vi "irrad calc color parameters.vi"(8 "error in (no error)":errorcluster, 10 "IRRAD Input Parameters":T1, 11 "Color Parameters in":T2) -> (0 "error out":errorcluster, 2 "IRRAD Input Parameters out":T1, 3 "Color Parameters out":T2)   [LabVIEW 2013, in "AvaSpec.lvlib" / "AVSirrad_support.lvlib"]
uses:
  AVSirrad_support.lvlib
  Acquisition/AvaSpec Color Parameters.ctl
  Acquisition/Sphere Indicator.ctl
  IRRAD input parameters.ctl
  Libraries/IRRAD-DLL/AVSirrad.lvlib
  AvaSpec.lvlib
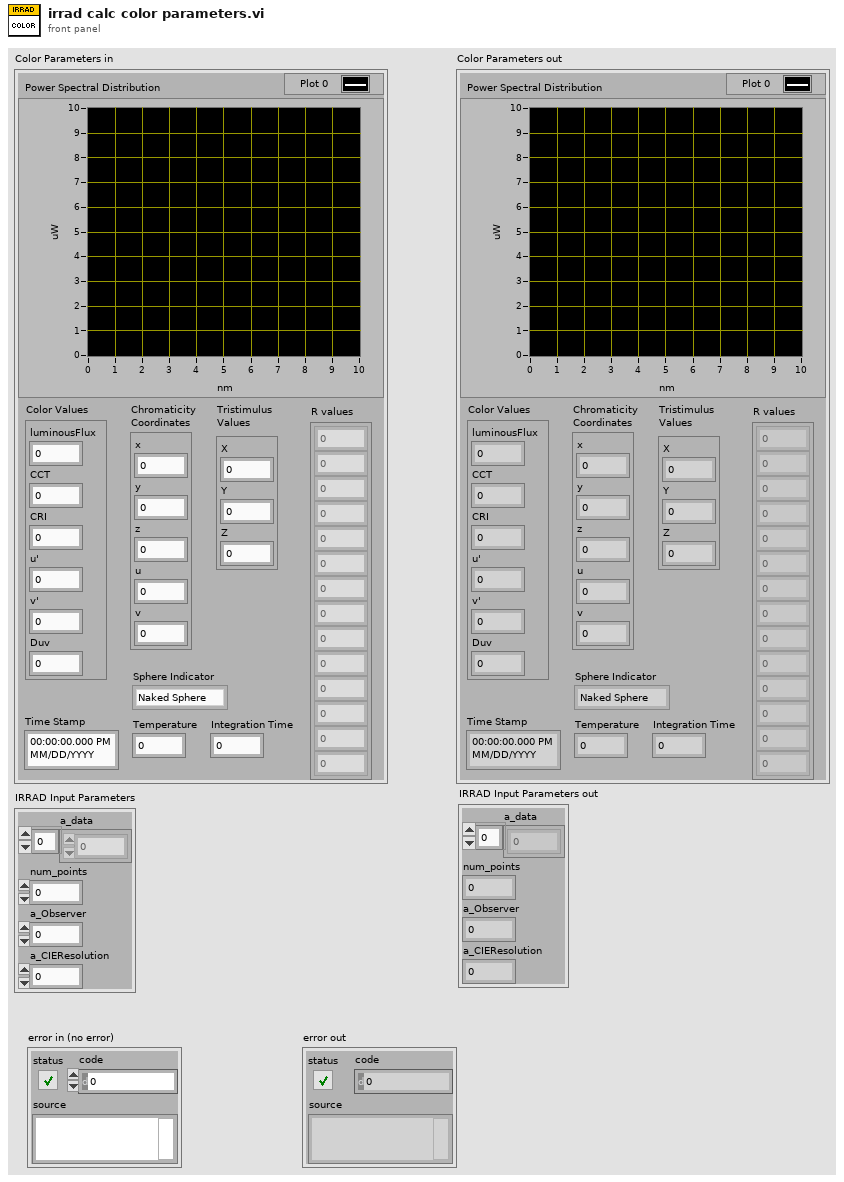
[diagram p1: front panel]
types:
  T1 = typedef "IRRAD input parameters.ctl" = cluster{"a_data":dbl[], "num_points":i32, "a_Observer":u8, "a_CIEResolution":u8}
  T2 = typedef "AvaSpec.lvlib/AvaSpec Color Parameters.ctl" = cluster{"Power Spectral Distribution":cluster{"X":dbl, "Y":dbl}[], "Color Values":cluster{"luminousFlux":dbl, "CCT":dbl, "CRI":dbl, "u'":dbl, "v'":dbl, "Duv":dbl}, "R values":dbl[], "Chromaticity \nCoordinates":cluster{"x":dbl, "y":dbl, "z":dbl, "u":dbl, "v":dbl}, "Tristimulus \nValues":cluster{"X":dbl, "Y":dbl, "Z":dbl}, "Time Stamp":timestamp, "Temperature":dbl, "Integration Time":dbl, "Sphere Indicator":T3}
  T3 = typedef "AvaSpec.lvlib/Sphere Indicator.ctl" = enum16{"Naked Sphere", "Insulated Sphere"}
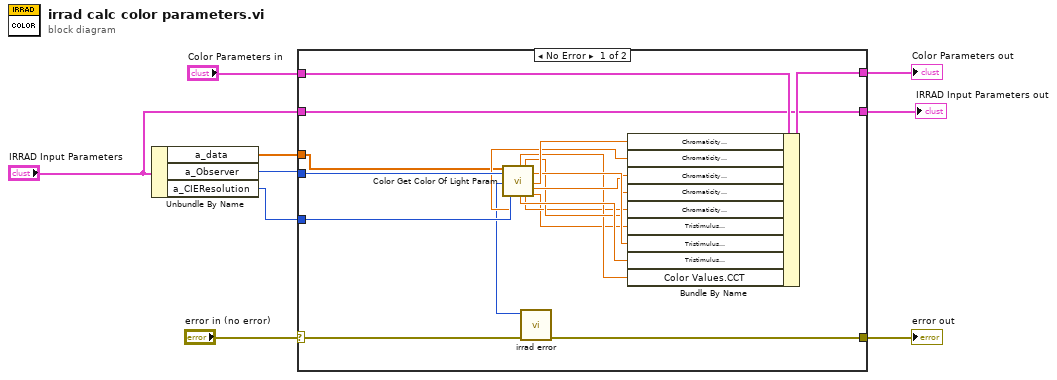
[diagram p0: block diagram]
diagram:
  n1 = Unbundle By Name("IRRAD Input Parameters") -> ("a_data"=w5:dbl[], "a_Observer"=w4:u8, "a_CIEResolution"=w3:u8)
  n2 = case shown="No Error" "error in (no error)" {
    selector: "error in (no error)" -> [w13 w30]
    tunnel: w4 -> [w27 _]
    tunnel: [w26 w30] -> w9
    tunnel: w3 -> [w25 _]
    tunnel: "Color Parameters in" -> [w24 w29]
    tunnel: [w23 w29] -> w7
    tunnel: w5 -> [w12 _]
    tunnel: "IRRAD Input Parameters" -> [w11 w28]
    tunnel: [w11 w28] -> w1
    frame No Error {
      n3 = call "Color Get Color Of Light Param.vi"("a_data"=w12, "a_Observer"=w27, "a_CIEResolution"=w25) -> ("function return"=w10:i16, "a_smally out"=w14:dbl, "a_Colortemperature out"=w17:dbl, "a_bigZ out"=w21:dbl, "a_u out"=w18:dbl, "a_v out"=w16:dbl, "a_bigY out"=w20:dbl, "a_smallx out"=w22:dbl, "a_smallz out"=w19:dbl, "a_bigX out"=w15:dbl)  [unwired: 5 in, 2 out]
      n4 = call "irrad error.vi"("error in (no error)"=w13, "Output Value"=w10) -> ("error out"=w26:errorcluster)  [unwired: 9 in]
      n5 = Bundle By Name(cluster=w24, "Chromaticity \nCoordinates.x"=w22, "Chromaticity \nCoordinates.y"=w14, "Chromaticity \nCoordinates.z"=w19, "Chromaticity \nCoordinates.u"=w18, "Chromaticity \nCoordinates.v"=w16, "Tristimulus \nValues.X"=w15, "Tristimulus \nValues.Y"=w20, "Tristimulus \nValues.Z"=w21, "Color Values.CCT"=w17) -> (w23:T2)
    }
    frame Error {
    }
  }
  "error out" <- w9
  "Color Parameters out" <- w7
  "IRRAD Input Parameters out" <- w1
